vi "read_attributes.vi"(8 "error in (no error)":errorcluster, 11 "BayesianGaussianMixture in":refnum<class "BayesianGaussianMixture.lvclass">) -> (0 "error out":errorcluster, 2 "attributes":T1, 3 "BayesianGaussianMixture out":refnum<class "BayesianGaussianMixture.lvclass">)   [LabVIEW 2020, in "BayesianGaussianMixture.lvclass"]
uses:
  BayesianGaussianMixture.lvclass
  Controls/bayesian_gaussian_mixture_attributes.ctl
  BayesianGaussianMixture.lvclass/BayesianGaussianMixture.ctl
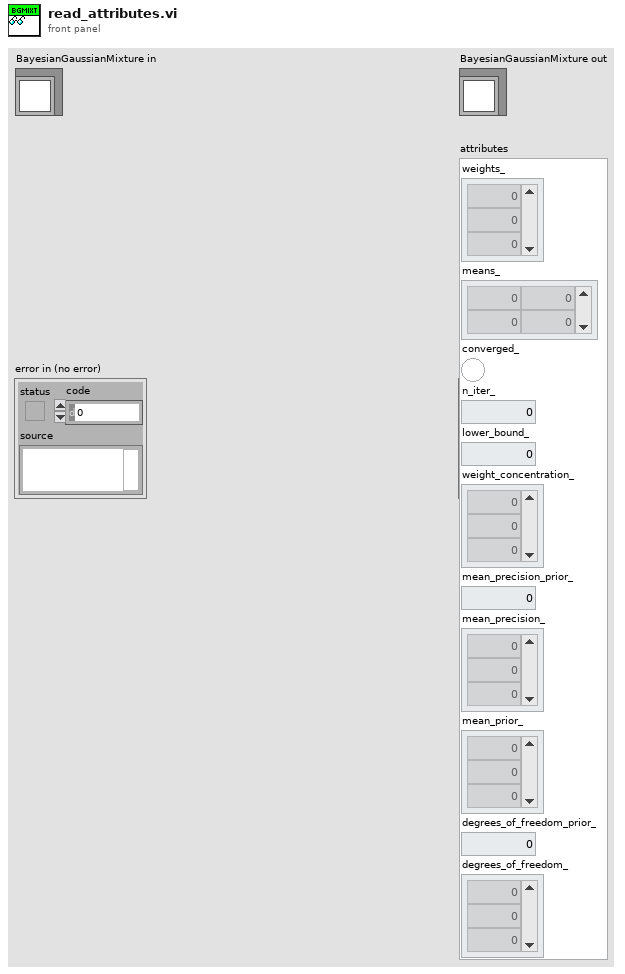
[diagram p1: front panel]
types:
  T1 = typedef "bayesian_gaussian_mixture_attributes.ctl" = cluster{"weights_":dbl[], "means_":dbl[][], "converged_":bool, "n_iter_":dbl, "lower_bound_":dbl, "weight_concentration_":dbl[][], "mean_precision_prior_":dbl, "mean_precision_":dbl[], "mean_prior_":dbl[], "degrees_of_freedom_prior_":dbl, "degrees_of_freedom_":dbl[]}
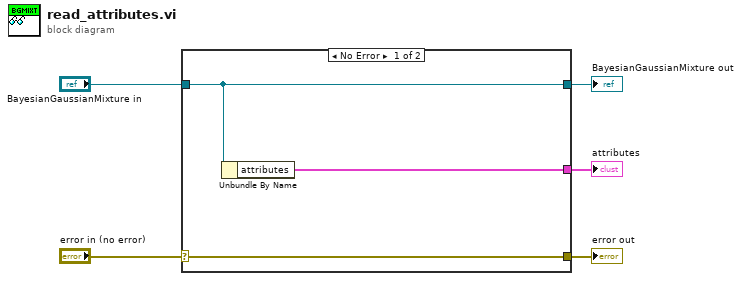
[diagram p0: block diagram]
diagram:
  n1 = case shown="No Error" "error in (no error)" {
    selector: "error in (no error)" -> [w8 w9]
    tunnel: [w8 w9] -> w4
    tunnel: [w7 w10] -> w2
    tunnel: "BayesianGaussianMixture in" -> [w7 w10]
    tunnel: [w6 _] -> w1
    frame No Error {
      n2 = Unbundle By Name(w7) -> ("attributes"=w6:T1)
    }
    frame Error {
    }
  }
  "error out" <- w4
  "BayesianGaussianMixture out" <- w2
  "attributes" <- w1
